vi "Dequeue.vi"(8 "error in (no error)":errorcluster, 11 "Sequencer Core in":refnum<class "Sequencer Core.lvclass">) -> (0 "error out":errorcluster, 1 "Message Priority":T1=enum."Normal", 2 "Message":refnum<class "Message.lvclass">, 3 "Sequencer Core out":refnum<class "Sequencer Core.lvclass">)   [LabVIEW 2020, in "Sequencer.lvlib" / "Sequencer Core.lvclass"]
doc: "Dequeue a message element from the Sequencer Core."
uses:
  Sequencer Core.lvclass
  PPL/HDH.Actor Framework.Core.Actor.lvlibp/1abvi3w/vi.lib/ActorFramework/Message Enqueuer/Message Priority.ctl
  PPL/HDH.Actor Framework.Core.Actor.lvlibp/1abvi3w/vi.lib/ActorFramework/Message/Message.lvclass
  Sequencer Core.lvclass/Sequencer Core.ctl
  Message Priority Queue/Message Priority Queue.lvclass
  PPL/HDH.Actor Framework.Core.Actor.lvlibp/1abvi3w/vi.lib/ActorFramework/Message Enqueuer/Message Enqueuer.lvclass
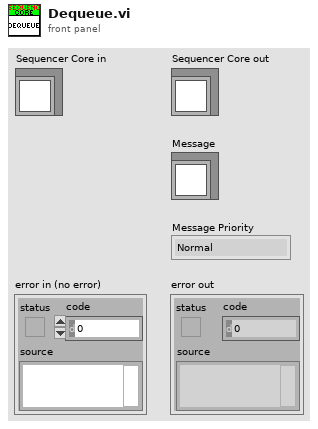
[diagram p1: front panel]
types:
  T1 = typedef "HDH.Actor Framework.Core.Actor.lvlibp/Message Enqueuer.lvclass/Message Priority.ctl" = enum16{"Low", "Normal", "High"}
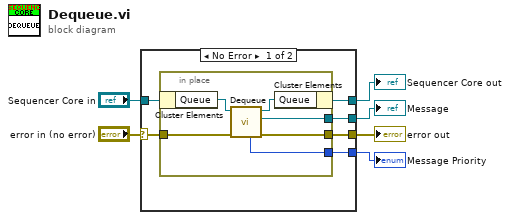
[diagram p0: block diagram]
diagram:
  n1 = case shown="No Error" "error in (no error)" {
    selector: "error in (no error)" -> [w11 w20]
    tunnel: [w10 w20] -> w5
    tunnel: [w7 w19] -> w3
    tunnel: "Sequencer Core in" -> [w12 w19]
    tunnel: [w9 _] -> w1
    tunnel: [w8 _] -> w2
    frame No Error {
      n2 = in-place {
        in-place-border: w11 -> [w16]
        in-place-border: [w15] -> w10
        in-place-border: [w14] -> w9
        in-place-border: [w13] -> w8
        n3 = in-place-cluster #1(w12) -> ("Queue"=w18:refnum<class "Message Priority Queue.lvclass">)
        n4 = call "Dequeue.vi"("error in (no error)"=w16, "Priority Queue in"=w18) -> ("error out"=w15:errorcluster, "element"=w14:refnum<class "Message.lvclass">, "Priority Queue out"=w17:refnum<class "Message Priority Queue.lvclass">, "priority"=w13:i32)  [unwired: 5 in, 1 out]
        n5 = in-place-cluster #1("Queue"=w17) -> (w7:refnum<class "Sequencer Core.lvclass">)
      }
    }
    frame Error {
    }
  }
  "error out" <- w5
  "Sequencer Core out" <- w3
  "Message Priority" <- w2
  "Message" <- w1
